vi "waveformGerneratorStickSlip_v3.vi"(0 "Ramp range":T4, 5 "Parameters":T1, 7 "InitialPositions":T2, 11 "Reset":cluster{"rampx":bool, "ustepx":bool}) -> (4 "DisplacementFinished":bool, 6 "MicroStepIndex":cluster{"CurrentUstep":i16, "NextUstep":i16}, 8 "RampIndex":cluster{"ramp index":i16, "NextRamp":i16}, 10 "Outputs":T3)   [LabVIEW 2016]
uses:
  <vilib>/rvi/FXPMathLib/FxpInterpret/XNode/nifxpmath_Interpret.xnode
  <vilib>/rvi/FXPMathLib/FxpMul/XNode/nifxpmath_Multiplier.xnode
  <vilib>/rvi/FXPMathLib/FxpSub/XNode/nifxpmath_Sub.xnode
  <instrlib>/_niInstr/Basic Elements/v1/FPGA/niInstr Basic Elements v1 FPGA.lvlib
  <vilib>/rvi/FXPMathLib/sim/FxpSim.dll
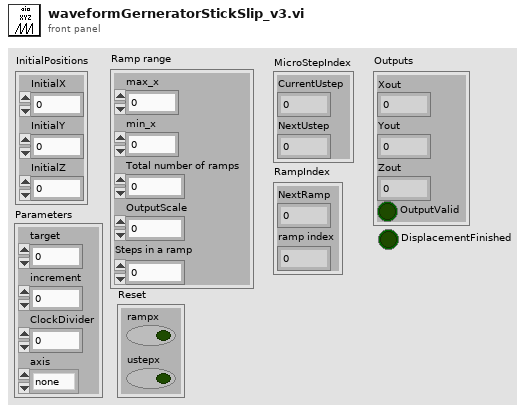
[diagram p1: front panel]
types:
  T1 = cluster{"target ":i16, "increment":i16, "ClockDivider":i16, "axis":enum16{"none", "x", "y", "z"}}
  T2 = cluster{"InitialX":fxp<+/-,16,16>, "InitialY":fxp<+/-,16,16>, "InitialZ":fxp<+/-,16,16>}
  T3 = cluster{"Xout":fxp<+/-,16,16>, "Yout":fxp<+/-,16,16>, "Zout":fxp<+/-,16,16>, "OutputValid":bool}
  T4 = cluster{"min_x":i16, "max_x":i16, "Total number of ramps":i16, "OutputScale":fxp<+/-,16,16>, "Steps in a ramp":i16}
  T5 = cluster{"InitialX":fxp<+/-,16,16>, "InitialY":fxp<+/-,16,16>, "InitialZ":fxp<+/-,16,16>, "output valid":bool}
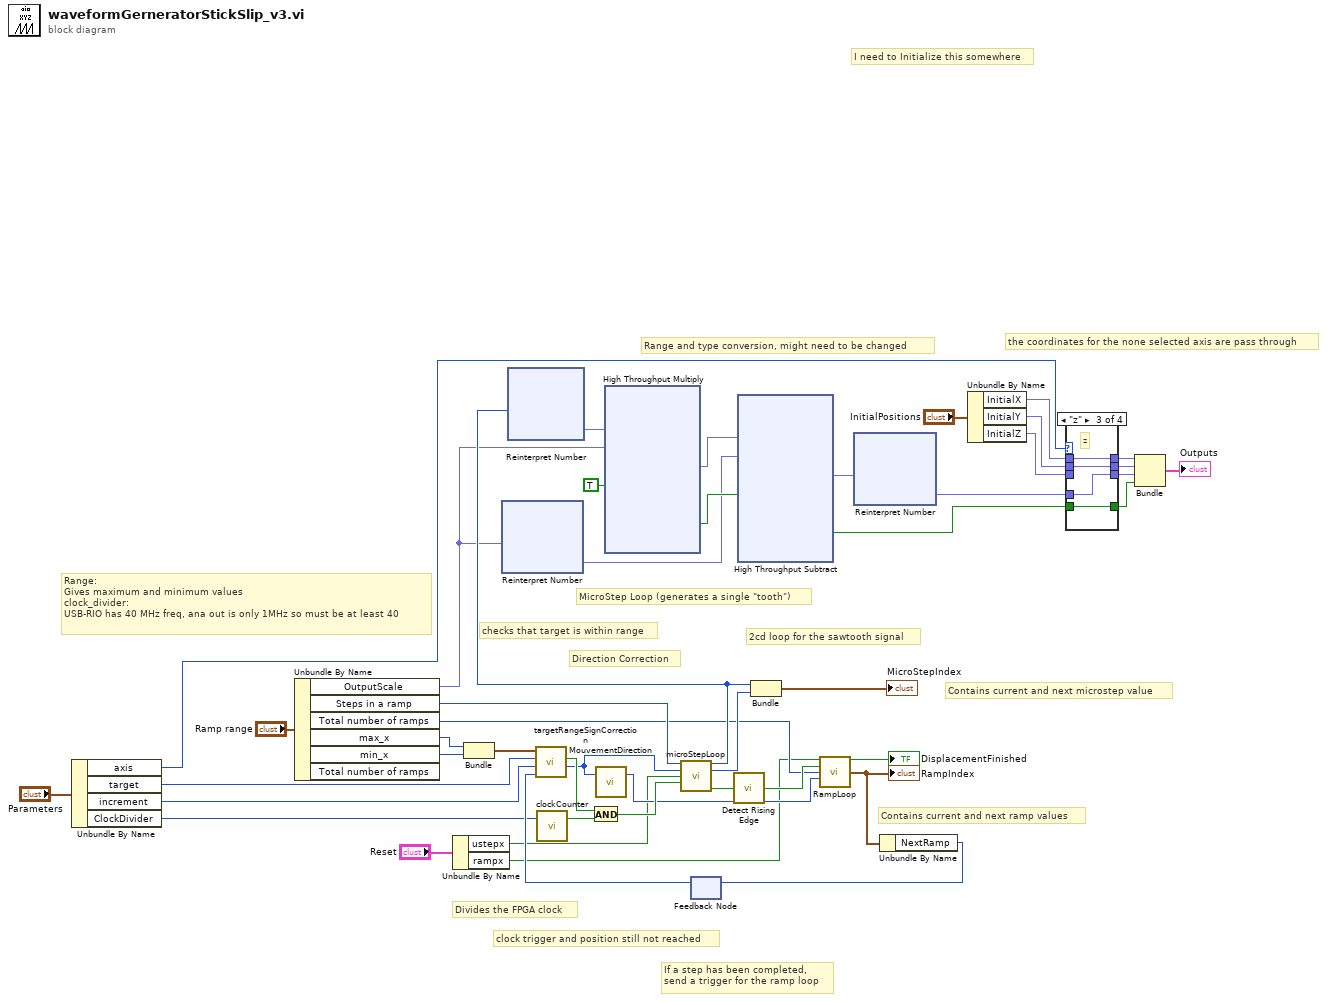
[diagram p0: block diagram]
diagram:
  # "I need to Initialize this somewhere"
  # "Range and type conversion, might need to be changed"
  # "the coordinates for the none selected axis are pass through"
  # "Contains current and next ramp values"
  # "Contains current and next microstep value"
  # "2cd loop for the sawtooth signal"
  # "MicroStep Loop (generates a single \"tooth\")"
  # "Direction Correction"
  # "checks that target is within range"
  # "Divides the FPGA clock"
  # "clock trigger and position still not reached"
  # "If a step has been completed, \nsend a trigger for the ramp loop"
  # "Range:\nGives maximum and minimum values\nclock_divider:\nUSB-RIO has 40 MHz freq, ana out is only 1MHz so must be at least 40"
  n1 = Unbundle By Name("Parameters") -> ("axis"=w5:enum16{"none", "x", "y", "z"}, "target"=w6:i16, "increment"=w7:i16, "ClockDivider"=w8:i16)
  n2 = Unbundle By Name("Ramp range") -> ("OutputScale"=w18:fxp<+/-,16,16>, "Steps in a ramp"=w19:i16, "Total number of ramps"=w17:i16, "max_x"=w21:i16, "min_x"=w20:i16)  [unwired: 1 out]
  n3 = Unbundle By Name("Reset") -> ("ustepx"=w14:bool, "rampx"=w15:bool)
  n4 = Bundle("max_x"=w21, "min_x"=w20) -> (w40:cluster{"max_x":i16, "min_x":i16})  [unwired: 1 in]
  n5 = xnode "Reinterpret Number"("x"=w18) -> ("y"=w31:fxp<+/-,16,4>)
  n6 = call "clockCounter.vi"("clock_divider_x"=w8) -> ("Clock"=w43:bool)  [unwired: 1 in, 1 out]
  n7 = feedback #1() -> (w44:i16)  [unwired: 1 in]
  n8 = call "targetRangeSignCorrection.vi"("Current Ramp Position"=w44, "increment_x"=w7, "target"=w6, "Ramp range"=w40) -> ("Increment corrected for direction"=w39:i16, "position not reached"=w42:bool)  [unwired: 1 in, 1 out]
  n9 = And(x=w42, y=w43) -> (x .and. y?=w41:bool)
  n10 = call "MouvementDirection.vi"("Increment corrected for direction"=w39) -> ("Mouvement Direction"=w38:i16)  [unwired: 1 in, 1 out]
  n11 = call "microStepLoop.vi"("StepsInAramp"=w19, "CorrectedIncrement"=w39, "ResetUstep"=w14, "Clock Trigger"=w41) -> ("CurrentUstep"=w34:i16, "NextUstep"=w37:i16, "TopRamp"=w46:bool)  [unwired: 7 in, 2 out]
  n12 = xnode "Reinterpret Number"("x"=w34) -> ("y"=w29:fxp<+/-,16,1>)
  n13 = xnode ("High Throughput Multiply")("x"=w29, "y"=w18, "input valid"=TRUE) -> ("x*y"=w32:fxp<+/-,16,16>, "output valid"=w33:bool)  [unwired: 1 in, 1 out]
  n14 = call <instrlib>:"Detect Rising Edge.vi"("signal"=w46) -> ("edge detected"=w45:bool)  [unwired: 14 in]
  n15 = xnode "High Throughput Subtract"("x"=w32, "y"=w31, "input valid"=w33) -> ("x-y"=w11:fxp<+/-,16,15>, "output valid"=w28:bool)  [unwired: 1 in, 1 out]
  n16 = Bundle("CurrentUstep"=w34, "NextUstep"=w37) -> (→"MicroStepIndex":cluster{"CurrentUstep":i16, "NextUstep":i16})  [unwired: 1 in]
  n17 = call "RampLoop.vi"("reset_ramp_x"=w15, "edge detected"=w45, "total number of ramps"=w17, "direction increment"=w38) -> ("DisplacementFinished"=→"DisplacementFinished":bool, "Ramp index"=w13:cluster{"ramp index":i16, "NextRamp":i16})  [unwired: 9 in, 1 out]
  "RampIndex" <- w13
  n18 = xnode "Reinterpret Number"("x"=w11) -> ("y"=w10:fxp<+/-,16,16>)
  n19 = Unbundle By Name(w13) -> ("NextRamp"=w12:i16)
  n20 = feedback-in #1(w12) -> ()
  n21 = Unbundle By Name("InitialPositions") -> ("InitialX"=w3:fxp<+/-,16,16>, "InitialY"=w2:fxp<+/-,16,16>, "InitialZ"=w1:fxp<+/-,16,16>)
  n22 = case shown="\"z\"" w5 {
    tunnel: w28 -> [w47 w51 w56 w59]
    tunnel: w10 -> [w48 w54 w55 _]
    tunnel: w3 -> [_ w53 w57 w62]
    tunnel: w2 -> [w50 _ w58 w61]
    tunnel: w1 -> [w49 w52 _ w60]
    tunnel: [w50 w54 w58 w61] -> w25
    tunnel: [w49 w52 w55 w60] -> w26
    tunnel: [w48 w53 w57 w62] -> w24
    tunnel: [w47 w51 w56 w59] -> w23
    frame "x" {
      # "x"
    }
    frame "y" {
      # "y"
    }
    frame "z" {
      # "z"
    }
    frame Default {
    }
  }
  n23 = Bundle("InitialX"=w24, "InitialY"=w25, "InitialZ"=w26, "output valid"=w23) -> (→"Outputs":T5)  [unwired: 1 in]
